vi "Split String Main.vi"(8 "error in":errorcluster, 10 "String In":string) -> (0 "error out":errorcluster, 2 "Formula Phrasing Binary Tree Out":refnum<class "Formula Phrasing Binary Tree Node.lvclass">)   [LabVIEW 2024, in "Formula String Spliter Library.lvlib"]
uses:
  Formula String Spliter Library.lvlib
  Formula Phrasing Binary Tree Node/Formula Phrasing Binary Tree Node.lvclass
  C:/Users/iio/Desktop/Bussiness/Tricorn Re/Madelbrot 4.0/General Library/Modules/Math Formula String Phrasing/Math Formula String Phrasing/Math Formula String Phrasing.lvclass
  Formula Phrasing Binary Tree Node/Formula Phrasing Binary Tree Node.lvclass/Formula Phrasing Binary Tree Node.ctl
  Formula Phrasing Binary Tree Node/Public Data/Write Left Child Node.vi
  Formula Phrasing Binary Tree Node/Public Data/Write Right Child Node.vi
  C:/Users/iio/Desktop/Bussiness/Tricorn Re/Madelbrot 4.0/General Library/Modules/Math Formula String Phrasing/Formula Phrasing Binary Tree Node/Formula Phrasing Binary Tree Node.lvclass
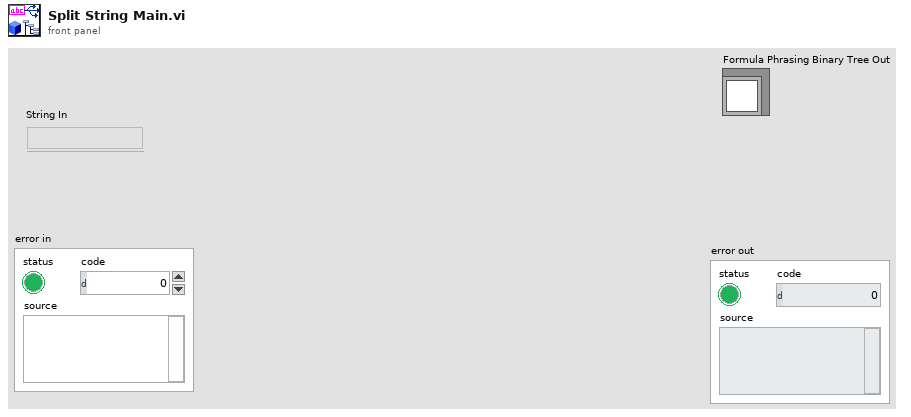
[diagram p1: front panel]
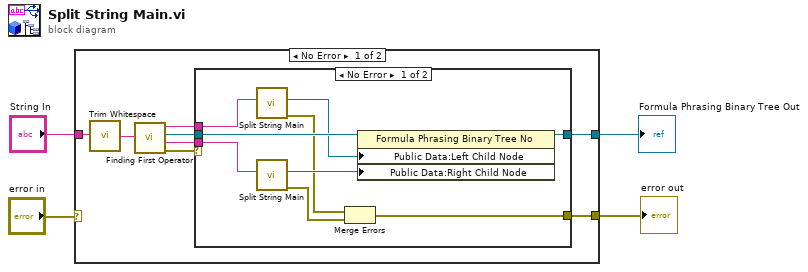
[diagram p0: block diagram]
diagram:
  n1 = case shown="No Error" "error in" {
    selector: "error in" -> [_ w23]
    tunnel: [w10 _] -> w4
    tunnel: "String In" -> [w9 _]
    tunnel: [w7 w23] -> w2
    frame No Error {
      n2 = call <vilib>:"Trim Whitespace.vi"("string"=w9) -> ("trimmed string"=w8:string)  [unwired: 1 in]
      n3 = call "Finding First Operator.vi"("String In"=w8) -> ("error out"=w5:errorcluster, "Right String Out"=w6:string, "First Operator Out"=w11:refnum<class "Formula Phrasing Binary Tree Node.lvclass">, "Left String Out"=w12:string)  [unwired: 7 in]
      n4 = case shown="No Error" w5 {
        selector: w5 -> [_ w22]
        tunnel: w12 -> [w21 _]
        tunnel: w11 -> [w20 _]
        tunnel: [w17 _] -> w10
        tunnel: [w14 w22] -> w7
        tunnel: w6 -> [w13 _]
        frame No Error {
          n5 = call "Split String Main.vi"("String In"=w21) -> ("error out"=w16:errorcluster, "Formula Phrasing Binary Tree Out"=w19:refnum<class "Formula Phrasing Binary Tree Node.lvclass">)  [unwired: 9 in]
          n6 = call "Split String Main.vi"("String In"=w13) -> ("error out"=w15:errorcluster, "Formula Phrasing Binary Tree Out"=w18:refnum<class "Formula Phrasing Binary Tree Node.lvclass">)  [unwired: 9 in]
          n7 = Merge Errors(w16, w15) -> (w14:errorcluster)
          n8 = property class="Formula Phrasing Binary Tree No"(reference=w20, "Public Data:Left Child Node"=w19, "Public Data:Right Child Node"=w18) -> (reference out=w17:refnum<class "Formula Phrasing Binary Tree Node.lvclass">)  [unwired: 1 in, 1 out]
        }
        frame Error {
        }
      }
    }
    frame Error {
    }
  }
  "Formula Phrasing Binary Tree Out" <- w4
  "error out" <- w2
